vi "Database adapter.vi"(8 "error in (no error)":errorcluster, 10 "function":enum16{"odczyt", "zapis"}(ring), 11 "Cluster":T2) -> (0 "error out":errorcluster, 1 "return code":i32, 3 "Boolean":bool)   [LabVIEW 2019]
doc: "This VI is responsible for saving license plate numbers in txt file and checking if license plates numbers are in our database. It`s actions depends on the name of fuction he recives on input."
uses:
  <vilib>/vision/Image Controls.llb/IMAQ Image.ctl
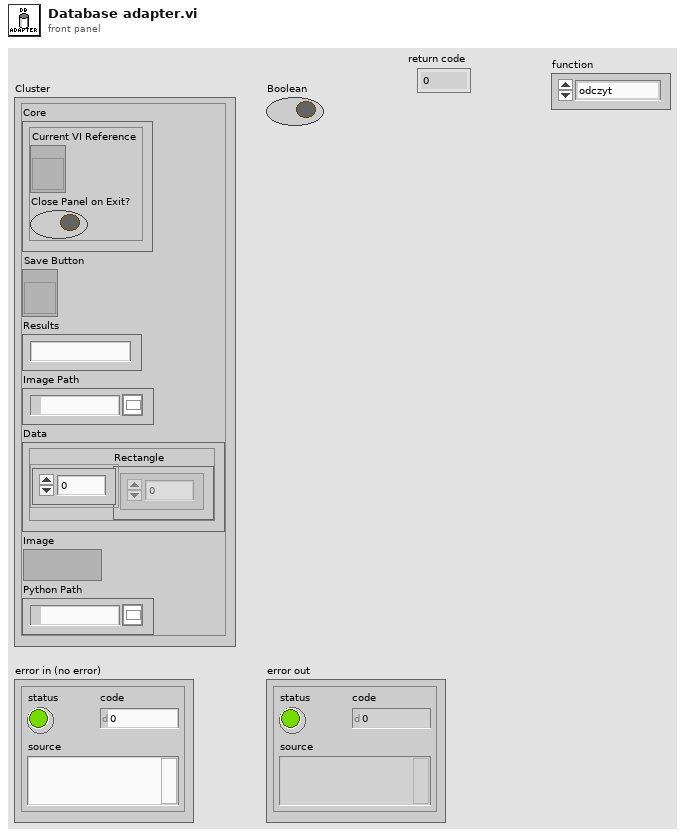
[diagram p1: front panel]
types:
  T1 = typedef "IMAQ Image.ctl" = refnum<image>
  T2 = cluster{"Core":cluster{"Current VI Reference":refnum<vi>, "Close Panel on Exit?":bool}, "Save Button":refnum<vi>, "Results":string, "Image Path":path, "Data":cluster{"Rectangle":i32[]}, "Image":T1, "Python Path":path}
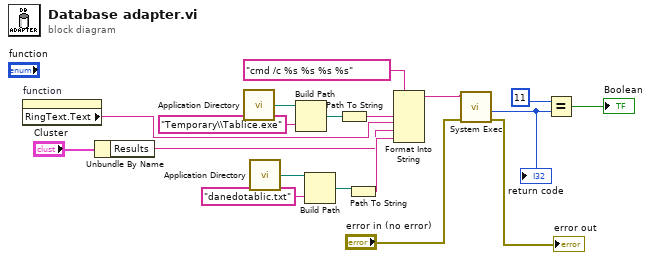
[diagram p0: block diagram]
diagram:
  n1 = property on="function" class="Enum (strict)"() -> ("RingText.Text"=w1:string)  [unwired: 2 in, 2 out]
  n2 = Unbundle By Name("Cluster") -> ("Results"=w2:string)
  n3 = call <vilib>:"Application Directory.vi"() -> ("Application Directory"=w10:path)
  n4 = call <vilib>:"Application Directory.vi"() -> ("Application Directory"=w13:path)
  n5 = Build Path ("Tablice exe")(base path=w10, name or relative path="Temporary\\Tablice.exe") -> (appended path=w12:path)
  n6 = Build Path ("Tablice exe")(base path=w13, name or relative path="danedotablic.txt") -> (appended path=w15:path)
  n7 = Path To String(path=w12) -> (string=w17:string)
  n8 = Path To String(path=w15) -> (string=w3:string)
  n9 = Format Into String(format string="cmd /c %s %s %s %s" ("command line"), w17, w1, w2, w3) -> (resulting string=w18:string)  [unwired: 2 in, 1 out]
  n10 = call <vilib>:"System Exec.vi"("error in (no error)"="error in (no error)", "command line"=w18) -> ("error out"=→"error out":errorcluster, "return code"=w7:i32)  [unwired: 6 in, 2 out]
  "return code" <- w7
  n11 = Equal?(x=11, y=w7) -> (x = y?=→"Boolean":bool)
